vi "Apply Brickwall Filter.vi"(8 "error in (no error)":errorcluster, 9 "Fs (Hz)":dbl=1.0 format="%#_13g", 10 "Signal In":dbl[](array[numeric]), 11 "Filter in":refnum<class "Filter.lvclass">) -> (0 "error out":errorcluster, 1 "Gain (dB)":dbl, 2 "Signal Out":dbl[](array[numeric]), 3 "Filter out":refnum<class "Filter.lvclass">)   [LabVIEW 2020, in "Filter.lvclass"]
uses:
  Filter.lvclass
  Filter.lvclass/Filter.ctl
  Utility VIs/Math VIs/FFT x(t) to dB,Degrees (1D).vi
  Utility VIs/Math VIs/Linear to dB (scalar).vi
  Utility VIs/Math VIs/Linear to dB (array).vi
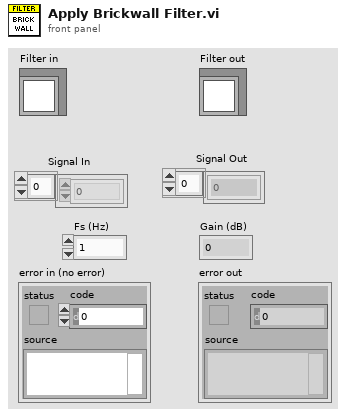
[diagram p1: front panel]
types:
  T1 = typedef "Filter.lvclass/Shape.ctl" = enum16{"OFF", "Lowpass", "Highpass", "Bandpass", "Bandstop"}
  T2 = typedef "Filter.lvclass/Units.ctl" = enum16{"Linear", "Octaves", "Min-Max"}
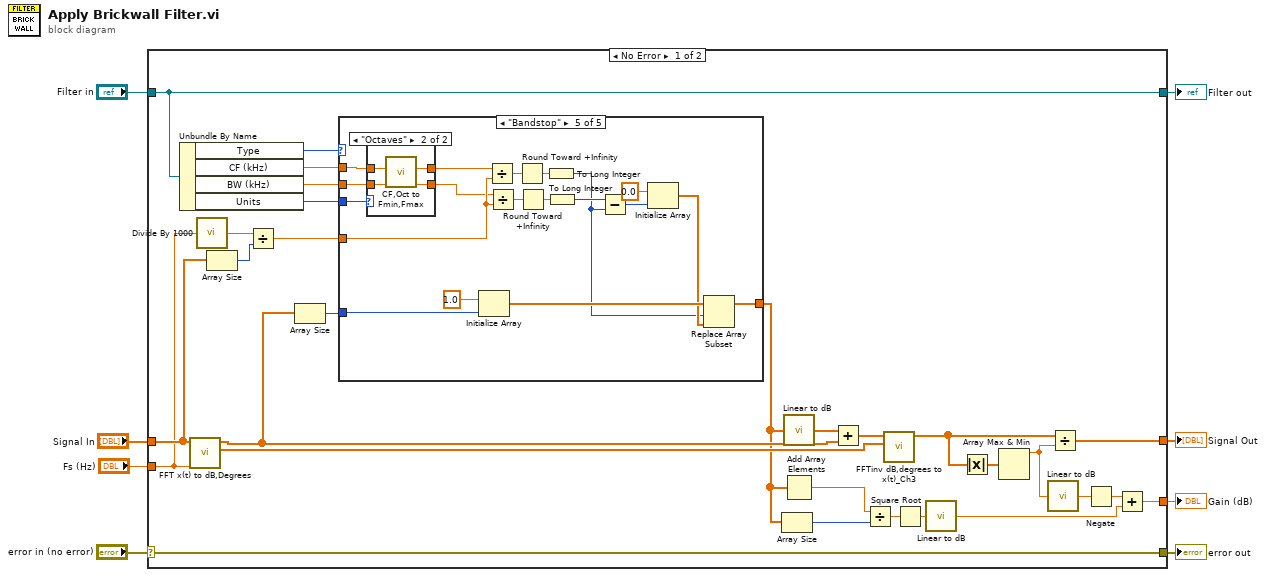
[diagram p0: block diagram]
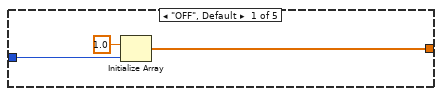
[diagram p2: hidden frame]
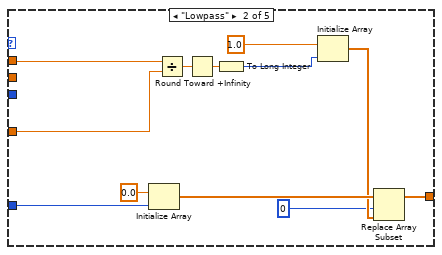
[diagram p3: hidden frame]
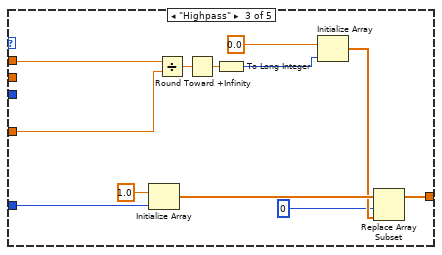
[diagram p4: hidden frame]
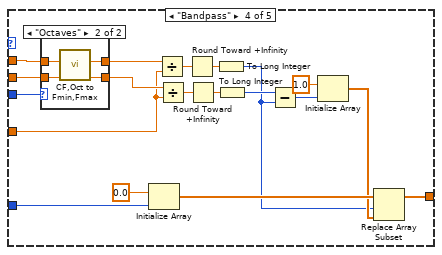
[diagram p5: hidden frame]
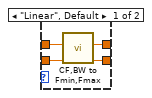
[diagram p6: hidden frame]
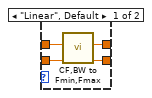
[diagram p7: hidden frame]
diagram:
  n1 = case shown="No Error" "error in (no error)" {
    selector: "error in (no error)" -> [w37 w120]
    tunnel: [w37 w120] -> w7
    tunnel: [w35 w119] -> w5
    tunnel: "Filter in" -> [w35 w119]
    tunnel: "Signal In" -> [w31 _]
    tunnel: [w24 _] -> w3
    tunnel: "Fs (Hz)" -> [w30 _]
    tunnel: [w17 _] -> w1
    frame No Error {
      n2 = Unbundle By Name(w35) -> ("Type"=w34:T1, "CF (kHz)"=w33:dbl, "BW (kHz)"=w32:dbl, "Units"=w26:T2)
      n3 = call-poly "FFT x(t) to dB,Degrees.vi"("Fs (Hz)"=w30, "X"=w31) -> ("+Freq Phase of FFT (degrees)"=w36:dbl[], "+Freq. Mag of FFT (dB rms)"=w15:dbl[])  [unwired: 7 in, 1 out]
      n4 = call "Divide By 1000.vi"("X"=w30) -> ("X/1000"=w27:dbl)
      n5 = Array Size(array=w31) -> (size(s)=w28:i32)
      n6 = Divide(x=w27, y=w28) -> (x/y=w29:dbl)
      n7 = Array Size(array=w15) -> (size(s)=w16:i32)
      n8 = case shown="\"Bandstop\"" w34 {
        tunnel: w16 -> [w40 w49 w61 w72 w103]
        tunnel: [w38 w47 w59 w70 w101] -> w9
        tunnel: w33 -> [_ w43 w55 w83 w96]
        tunnel: w32 -> [_ _ _ w82 w95]
        tunnel: w29 -> [_ w41 w53 w75 w106]
        tunnel: w26 -> [_ _ _ w65 w94]
        frame "OFF", Default {
          n9 = Initialize Array(1.0 ("element"), w40) -> (w38:dbl[])
        }
        frame "Lowpass" {
          n10 = Initialize Array(0.0 ("element"), w49) -> (w48:dbl[])
          n11 = Divide(x=w43, y=w41) -> (x/y=w51:dbl)
          n12 = Round Toward +Infinity(x=w51) -> (ceil(x): smallest int >= x=w52:dbl)
          n13 = To Long Integer(number=w52) -> (32bit integer=w44:i32)
          n14 = Initialize Array(1.0 ("element"), w44) -> (w45:dbl[])
          n15 = Replace Array Subset(array=w48, new element=w45, index=0) -> (w47:dbl[])
        }
        frame "Highpass" {
          n16 = Initialize Array(1.0 ("element"), w61) -> (w60:dbl[])
          n17 = Divide(x=w55, y=w53) -> (x/y=w63:dbl)
          n18 = Round Toward +Infinity(x=w63) -> (ceil(x): smallest int >= x=w64:dbl)
          n19 = To Long Integer(number=w64) -> (32bit integer=w56:i32)
          n20 = Initialize Array(0.0 ("element"), w56) -> (w57:dbl[])
          n21 = Replace Array Subset(array=w60, new element=w57, index=0) -> (w59:dbl[])
        }
        frame "Bandpass" {
          n22 = case shown="\"Octaves\"" w65 {
            tunnel: w83 -> [w87 w91]
            tunnel: w82 -> [w86 w90]
            tunnel: [w85 w89] -> w79
            tunnel: [w84 w88] -> w76
            frame "Linear", Default {
              n23 = call "CF,BW to Fmin,Fmax.vi"("BW"=w86, "CF"=w87) -> ("Fmax"=w84:dbl, "Fmin"=w85:dbl)  [unwired: 8 in]
            }
            frame "Octaves" {
              n24 = call "CF,Oct to Fmin,Fmax.vi"("BW"=w90, "CF"=w91) -> ("Fmax"=w88:dbl, "Fmin"=w89:dbl)  [unwired: 8 in]
            }
          }
          n25 = Initialize Array(0.0 ("element"), w72) -> (w71:dbl[])
          n26 = Divide(x=w79, y=w75) -> (x/y=w80:dbl)
          n27 = Divide(x=w76, y=w75) -> (x/y=w77:dbl)
          n28 = Round Toward +Infinity(x=w80) -> (ceil(x): smallest int >= x=w81:dbl)
          n29 = Round Toward +Infinity(x=w77) -> (ceil(x): smallest int >= x=w78:dbl)
          n30 = To Long Integer(number=w81) -> (32bit integer=w66:i32)
          n31 = To Long Integer(number=w78) -> (32bit integer=w74:i32)
          n32 = Subtract(x=w74, y=w66) -> (x-y=w69:i32)
          n33 = Initialize Array(1.0 ("element"), w69) -> (w67:dbl[])
          n34 = Replace Array Subset(array=w71, new element=w67, index=w66) -> (w70:dbl[])
        }
        frame "Bandstop" {
          n35 = case shown="\"Octaves\"" w94 {
            tunnel: w96 -> [w114 w118]
            tunnel: w95 -> [w113 w117]
            tunnel: [w112 w116] -> w93
            tunnel: [w111 w115] -> w92
            frame "Linear", Default {
              n36 = call "CF,BW to Fmin,Fmax.vi"("BW"=w113, "CF"=w114) -> ("Fmax"=w111:dbl, "Fmin"=w112:dbl)  [unwired: 8 in]
            }
            frame "Octaves" {
              n37 = call "CF,Oct to Fmin,Fmax.vi"("BW"=w117, "CF"=w118) -> ("Fmax"=w115:dbl, "Fmin"=w116:dbl)  [unwired: 8 in]
            }
          }
          n38 = Initialize Array(1.0 ("element"), w103) -> (w102:dbl[])
          n39 = Divide(x=w93, y=w106) -> (x/y=w109:dbl)
          n40 = Divide(x=w92, y=w106) -> (x/y=w107:dbl)
          n41 = Round Toward +Infinity(x=w109) -> (ceil(x): smallest int >= x=w110:dbl)
          n42 = Round Toward +Infinity(x=w107) -> (ceil(x): smallest int >= x=w108:dbl)
          n43 = To Long Integer(number=w110) -> (32bit integer=w97:i32)
          n44 = To Long Integer(number=w108) -> (32bit integer=w105:i32)
          n45 = Subtract(x=w105, y=w97) -> (x-y=w100:i32)
          n46 = Initialize Array(0.0 ("element"), w100) -> (w98:dbl[])
          n47 = Replace Array Subset(array=w102, new element=w98, index=w97) -> (w101:dbl[])
        }
      }
      n48 = Array Size(array=w9) -> (size(s)=w11:i32)
      n49 = call-poly "Linear to dB.vi"("linear"=w9) -> ("dB"=w14:dbl[])
      n50 = Add Array Elements(numeric array=w9) -> (sum=w10:dbl)
      n51 = Add(x=w14, y=w15) -> (x+y=w19:dbl[])
      n52 = Divide(x=w10, y=w11) -> (x/y=w12:dbl)
      n53 = call "FFTinv dB,degrees to x(t)_Ch3.vi"("+Freq Phase of FFT (degrees)"=w36, "+Freq. Mag of FFT (rms dB)"=w19) -> ("X(t)"=w23:dbl[])  [unwired: 8 in, 1 out]
      n54 = Square Root(x=w12) -> (sqrt(x)=w18:dbl)
      n55 = call-poly "Linear to dB.vi"("Linear"=w18) -> ("dB"=w13:dbl)
      n56 = Absolute Value(x=w23) -> (abs(x)=w25:dbl[])
      n57 = Array Max & Min(array=w25) -> (max value=w22:dbl)  [unwired: 3 out]
      n58 = call-poly "Linear to dB.vi"("Linear"=w22) -> ("dB"=w21:dbl)
      n59 = Divide(x=w23, y=w22) -> (x/y=w24:dbl[])
      n60 = Negate(x=w21) -> (-x=w20:dbl)
      n61 = Add(x=w20, y=w13) -> (x+y=w17:dbl)
    }
    frame Error {
    }
  }
  "error out" <- w7
  "Filter out" <- w5
  "Signal Out" <- w3
  "Gain (dB)" <- w1
